vi "Get Value by Array (Numeric Value).vi"(8 "error in (no error)":errorcluster, 10 "Keys":string[](array[string]), 11 "JSON Object in":refnum<class "JSON Object.lvclass">) -> (0 "error out":errorcluster, 2 "value":dbl)   [LabVIEW 2016, in "LVJSON.lvlib" / "JSON Object.lvclass"]
uses:
  JSON Object.lvclass
  Get Value by Array (Numeric).vi
  JSON Numeric/Read value (Numeric).vi
  JSON Basic Type/JSON Literal.lvclass
  JSON Numeric/JSON Numeric.lvclass
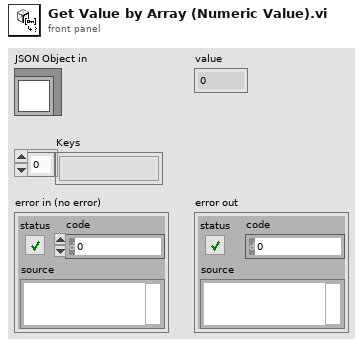
[diagram p1: front panel]
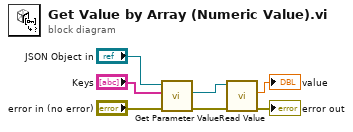
[diagram p0: block diagram]
diagram:
  n1 = call-poly "Get Parameter Value.vi"("error in (no error)"="error in (no error)", "Keys"="Keys", "JSON Object in"="JSON Object in") -> ("error out"=w4:errorcluster, "JSON Numeric out"=w1:refnum<class "JSON Numeric.lvclass">)  [unwired: 7 in]
  n2 = call-poly "Read Value.vi"("error in (no error)"=w4, "JSON Numeric in"=w1) -> ("error out"=→"error out":errorcluster, "value"=→"value":dbl)  [unwired: 8 in]
